vi "Spectrogram Global.vi"() -> ()   [LabVIEW 2023, in "Spectrogram.lvlib" / "Spectrogram.lvclass"]
uses:
  Spectrogram.lvclass
panel:
  in  "Color Table Values":u16[](array[ring])=[0, 1, 2, 3, 4, 5] items=["Rainbow", "Inverse gray", "Gray", "Color table 1", "Color table 2", "Color table 3"]
  in  "Color Table Strings":string[](array[string])=["Rainbow", "Inverse gray", "Gray", "Color table 1", "Color table 2", "Color table 3"]
  in  "Color Table":string="Color Table"
  in  "Length":string="Length"
  in  "Type Values":i32[](array[ring])=[0, 1, 2, 3, 4, 5, 6, 7, 8, 9, 10] items=["None ", "Hanning", "Hamming", "Blackman-Harris", "Exact Blackman", "Blackman", "Flat Top", "4 Term B-Harris ", "7 Term B-Harris", "Low Sidelobe", "Gaussian"]
  in  "Type Strings":string[](array[string])=["None", "Hanning", "Hamming", "Blackman-Harris", "Exact Blackman", "Blackman", "Flat Top", "4 Term B-Harris", "7 Term B-Harris", "Low Sidelobe", "Gaussian"]
  in  "Type":string="Type"
  in  "Frequency bins":string="Frequency bins"
  in  "Time steps":string="Time steps"
  in  "Extension Values":u16[](array[ring])=[0, 1, 2] items=["Zero padding", "Symmetric", "Periodic"]
  in  "Extension Strings":string[](array[string])=["Zero padding", "Symmetric", "Periodic"]
  in  "Extension":string="Extension"
  in  "Show Spectrogram Window":string="Show Spectrogram Window"
  in  "Select Channel":string="Select Channel"
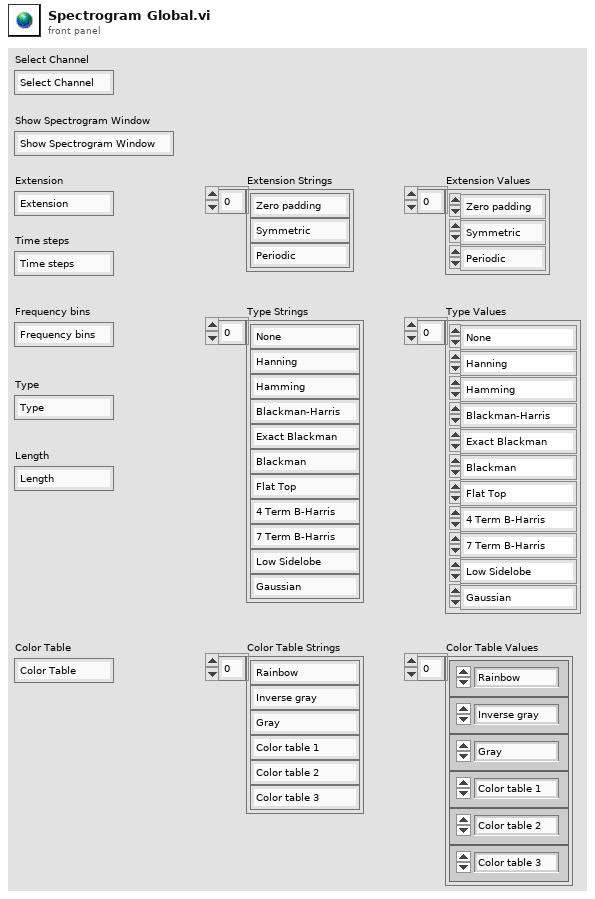
[diagram p1: front panel]
diagram:
